vi "highlight_table_cells.vi"(10 "Limit fail":bool[][](array[boolean]), 11 "Table in":refnum<vi>) -> (3 "Some limit fail":bool)   [LabVIEW 2013]
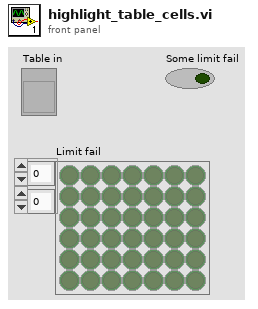
[diagram p1: front panel]
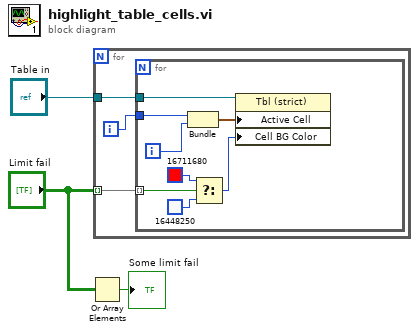
[diagram p0: block diagram]
diagram:
  n1 = Or Array Elements(Boolean array="Limit fail") -> (logical OR=→"Some limit fail":bool)
  n2 = for {
    tunnel: "Table in" -> [w6]
    tunnel: "Limit fail" -> [w4] mode=indexing
    i -> [w5]
    n3 = for {
      tunnel: w6 -> [w14]
      tunnel: w5 -> [w13]
      tunnel: w4 -> [w10] mode=indexing
      i -> [w12]
      n4 = Bundle(w13, w12) -> (w11:cluster{i32, i32})  [unwired: 1 in]
      n5 = Select(t=u32 16711680, s=w10, f=u32 16448250) -> (s? t:f=w7:u32)
      n6 = property class="Tbl (strict)"(reference=w14, "Active Cell"=w11, "Cell BG Color"=w7) -> ()  [unwired: 1 in, 2 out]
    }
  }
